vi "Calculate-temperature-statistics.vi"(11 "Temperature array":dbl[](array[numeric])) -> (3 "Temperature characteristics":T1 {"Stand. dev. temperature" format="%#.1f"; "Min. temperature" format="%#.0f"; "Max. temperature" format="%#.0f"; "Average temperature" format="%#.0f"})   [LabVIEW 2013, in "CameraVision.lvlib" / "CV-Temperature.lvclass"]
uses:
  CV-Temperature.lvclass
  Temperature-characteristics.ctl
  <vilib>/Analysis/NI_AALBase.lvlib
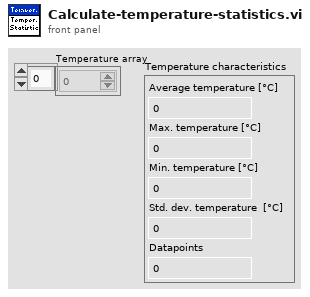
[diagram p1: front panel]
types:
  T1 = typedef "CameraVision.lvlib/CV-Temperature.lvclass/Temperature-characteristics.ctl" = cluster{"Average temperature ":dbl, "Max. temperature":dbl, "Min. temperature":dbl, "Stand. dev. temperature":dbl, "Datapoints":dbl}
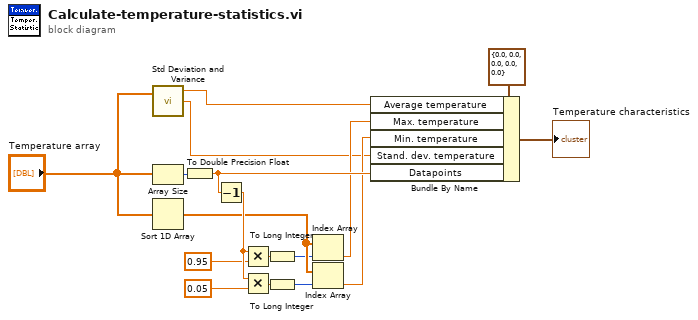
[diagram p0: block diagram]
diagram:
  n1 = call <vilib>:"Std Deviation and Variance.vi"("X"="Temperature array") -> ("mean"=w2:dbl, "standard deviation"=w3:dbl)  [unwired: 1 in, 1 out]
  n2 = Array Size(array="Temperature array") -> (size(s)=w4:i32)
  n3 = Sort 1D Array(array="Temperature array") -> (sorted array=w13:dbl[])
  n4 = To Double Precision Float(number=w4) -> (double precision float=w16:dbl)
  n5 = Decrement(x=w16) -> (x-1=w17:dbl)
  n6 = Multiply(x=w17, y=0.95) -> (x*y=w8:dbl)
  n7 = Multiply(x=w17, y=0.05) -> (x*y=w11:dbl)
  n8 = To Long Integer(number=w8) -> (32bit integer=w10:i32)
  n9 = To Long Integer(number=w11) -> (32bit integer=w12:i32)
  n10 = Index Array(array=w13, index=w10) -> (element=w14:dbl)
  n11 = Index Array(array=w13, index=w12) -> (element=w15:dbl)
  n12 = Bundle By Name(cluster=T1 {"Average temperature "=0.0, "Max. temperature"=0.0, "Min. temperature"=0.0, "Stand. dev. temperature"=0.0, "Datapoints"=0.0} ("Temperature characteristics"), "Average temperature"=w2, "Max. temperature"=w14, "Min. temperature"=w15, "Stand. dev. temperature"=w3, "Datapoints"=w16) -> (→"Temperature characteristics":T1)
